vi "Wavelength Range (YJ 20190220).vi"() -> ()   [LabVIEW 2017]
panel:
  out "WL Range":dbl[](array[numeric])
  in  "Step size (nm)":sgl=5.0 min=1 step=0.1
  in  "End Wavelength (nm)":dbl=1000.0 min=250.0 max=1350.0 step=0.1
  in  "Start Wavelength (nm)":dbl=350.0 min=250.0 max=1200.0 step=0.1
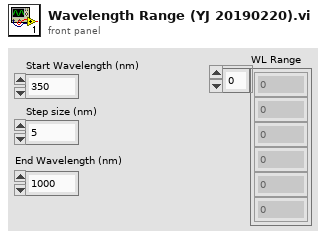
[diagram p1: front panel]
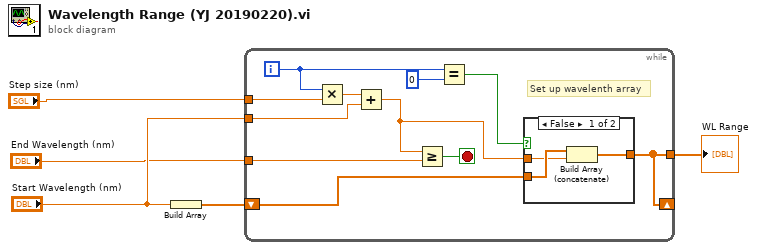
[diagram p0: block diagram]
diagram:
  n1 = Build Array "Build Array"("Start Wavelength (nm)") -> (w5:dbl[])
  n2 = while {
    shift-right: [w6] -> _
    shift-left: w5 -> [w8]
    tunnel: "Step size (nm)" -> [w15]
    tunnel: "End Wavelength (nm)" -> [w16]
    tunnel: "Start Wavelength (nm)" -> [w9]
    tunnel: [w6] -> w1
    i -> [w11]
    stop <- w13 stop-if-true
    # "Set up wavelenth array"
    n3 = Multiply(x=w11, y=w15) -> (x*y=w14:sgl)
    n4 = Add(x=w14, y=w9) -> (x+y=w7:dbl)
    n5 = Greater Or Equal?(x=w7, y=w16) -> (x >= y?=w13:bool)
    n6 = Equal?(x=w11, y=0) -> (x = y?=w10:bool)
    n7 = case shown="False" w10 {
      tunnel: w8 -> [w19 w20]
      tunnel: w7 -> [w18 _]
      tunnel: [w17 w20] -> w6
      frame False {
        n8 = Build Array (concatenate)(w19, w18) -> (w17:dbl[])
      }
      frame True {
      }
    }
  }
  "WL Range" <- w1
